vi "oauth2_authorize_pkce.vi"(6 "redirect_uri":string, 8 "error in (no error)":errorcluster, 9 "code_challenege_method":T1=enum."sha256", 10 "code_verifier":string, 11 "client_id":string) -> (0 "error out":errorcluster, 3 "auth_url":string)   [LabVIEW 2015, in "lv-dropbox.lvlib"]
uses:
  lv-dropbox.lvlib
  _controls/code_challenge_method.ctl
  private/cryptography/cryptography.lvlib
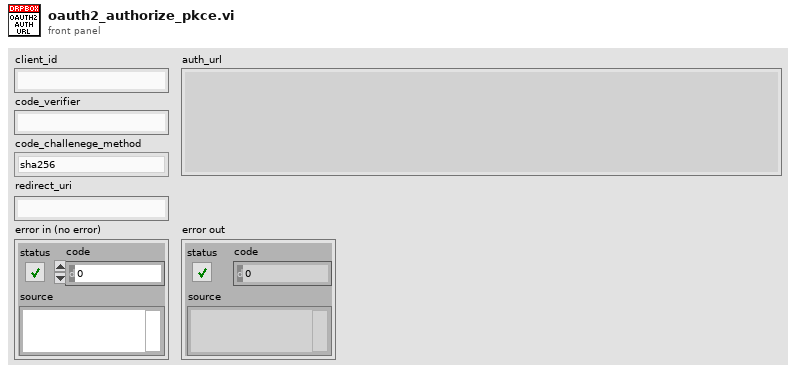
[diagram p1: front panel]
types:
  T1 = typedef "lv-dropbox.lvlib/code_challenge_method.ctl" = enum16{"<challenge_method>", "plain", "sha256"}
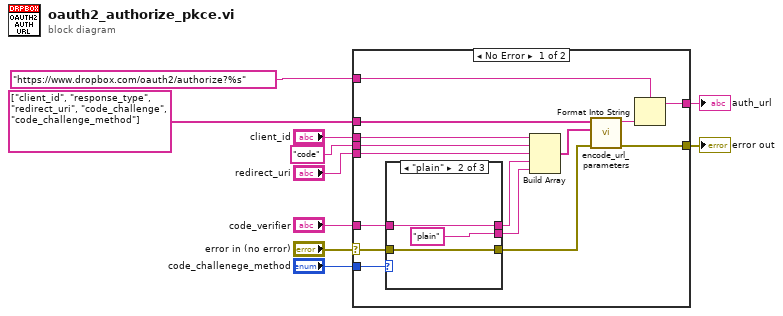
[diagram p0: block diagram]
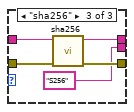
[diagram p3: hidden frame]
diagram:
  n1 = case shown="No Error" "error in (no error)" {
    selector: "error in (no error)" -> [w24 w35]
    tunnel: [w20 w35] -> w8
    tunnel: "https://www.dropbox.com/oauth2/authorize?%s" ("url") -> [w21 _]
    tunnel: "client_id" -> [w16 _]
    tunnel: "code_verifier" -> [w25 _]
    tunnel: [w23 _] -> w5
    tunnel: "code_challenege_method" -> [w22 _]
    tunnel: string[] ["client_id", "response_type", "redirect_uri", "code_challenge", "code_challenge_method"] -> [w17 _]
    tunnel: "code" -> [w14 _]
    tunnel: "redirect_uri" -> [w13 _]
    frame No Error {
      n2 = case shown="\"plain\"" w22 {
        tunnel: [_ w29 w34] -> w12
        tunnel: w25 -> [_ w29 w33]
        tunnel: w24 -> [w26 w28 w32]
        tunnel: [w26 w28 w31] -> w19
        tunnel: [_ "plain" ("url") "S256" ("url")] -> w11
        frame Default {
        }
        frame "plain" {
        }
        frame "sha256" {
          n3 = call "sha256.vi"("error in (no error)"=w32, "data_decoded"=w33) -> ("error out"=w31:errorcluster, "data_encoded"=w34:string)  [unwired: 8 in]
        }
      }
      n4 = Build Array(w16, w14, w13, w12, w11) -> (w15:string[])
      n5 = call "encode_url_parameters.vi"("error in (no error)"=w19, "value []"=w15, "key []"=w17) -> ("error out"=w20:errorcluster, "url_encoded_string"=w18:string)  [unwired: 7 in]
      n6 = Format Into String(format string=w21, w18) -> (resulting string=w23:string)  [unwired: 2 in, 1 out]
    }
    frame Error {
    }
  }
  "error out" <- w8
  "auth_url" <- w5
